vi "controlOutput.vi"(7 "Set":bool, 8 "error in":errorcluster, 9 "enable output in":bool=TRUE, 10 "axis in":u8, 11 "connection ID":refnum<k5>) -> (0 "error out":errorcluster, 1 "enable output out":bool=TRUE, 2 "axis out":u8, 3 "connection ID":refnum<k5>)   [LabVIEW 2019]
panel:
  in  "Set Command":string="com.attocube.amc.control.setControlOutput"
  in  "Get Command":string="com.attocube.amc.control.getControlOutput"
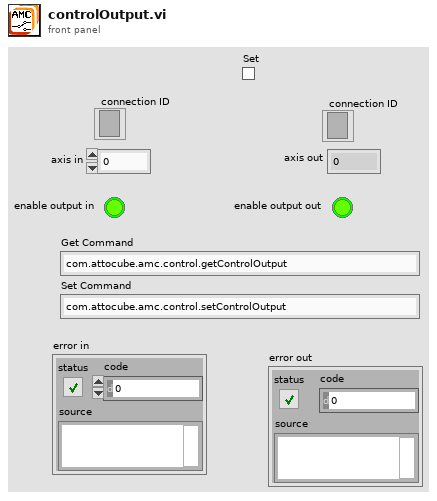
[diagram p1: front panel]
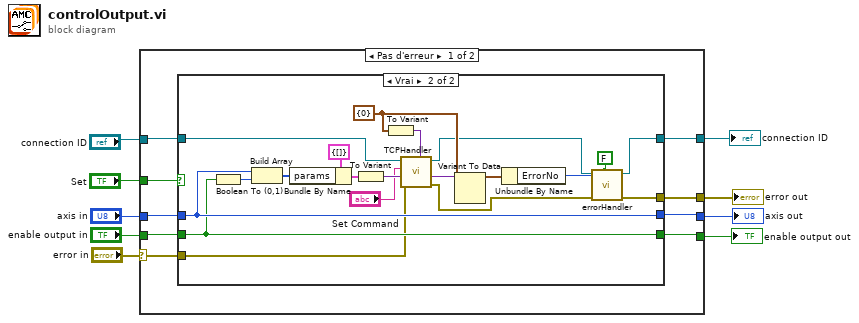
[diagram p0: block diagram]
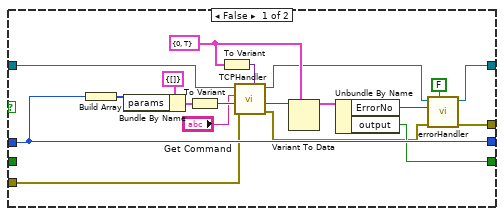
[diagram p2: hidden frame]
diagram:
  n1 = case shown="Pas d'erreur" "error in" {
    selector: "error in" -> [w10 w61]
    tunnel: "axis in" -> [w16 w59]
    tunnel: [w11 w61] -> w1
    tunnel: [w15 w59] -> w8
    tunnel: "Set" -> [w12 _]
    tunnel: [w13 w60] -> w6
    tunnel: "enable output in" -> [w14 w60]
    tunnel: [w18 w58] -> w4
    tunnel: "connection ID" -> [w17 w58]
    frame No Error {
      n2 = case shown="Vrai" w12 {
        tunnel: [w22 w41] -> w18
        tunnel: w17 -> [w27 w51]
        tunnel: w16 -> [w29 w49]
        tunnel: [w29 w49] -> w15
        tunnel: [w26 w48] -> w13
        tunnel: w14 -> [_ w48]
        tunnel: [w28 w45] -> w11
        tunnel: w10 -> [w20 w38]
        frame False {
          w24 = cluster{"ErrorNo":i16, "output":bool} {"ErrorNo"=0, "output"=TRUE} ("input cluster")
          n3 = Build Array(w29) -> (w33:u8[])
          n4 = Bundle By Name(cluster=cluster{"params":i32[]} {"params"=[]} ("input cluster"), "params"=w33) -> (w34:cluster{"params":i32[]})
          n5 = To Variant(anything=w34) -> (Variant=w35:variant)
          n6 = To Variant(anything=w24) -> (Variant=w25:variant)
          n7 = call <userlib>:"TCPHandler.vi"("result Types"=w25, "error in (no error)"=w20, "params"=w35, "method"="Get Command", "connection ID"=w27) -> ("error out"=w19:errorcluster, "result"=w31:variant, "connection ID"=w23:refnum<k5>)  [unwired: 3 in, 1 out]
          n8 = Variant To Data(type=w24, Variant=w31) -> (data=w36:cluster{"ErrorNo":i16, "output":bool})  [unwired: 1 in, 1 out]
          n9 = Unbundle By Name(w36) -> ("ErrorNo"=w37:i16, "output"=w26:bool)
          n10 = call <userlib>:"errorHandler.vi"("show popup"=FALSE, "error in"=w19, "error number"=w37, "connection ID"=w23) -> ("error out"=w28:errorcluster, "connection ID"=w22:refnum<k5>)  [unwired: 6 in]
        }
        frame True {
          w43 = cluster{"ErrorNo":i16} {"ErrorNo"=0} ("input cluster")
          n11 = Boolean To (0,1)(Boolean=w48) -> (0, 1=w55:i16)
          n12 = Build Array(w49, w55) -> (w53:i16[])
          n13 = Bundle By Name(cluster=cluster{"params":i32[]} {"params"=[]} ("input cluster"), "params"=w53) -> (w52:cluster{"params":i32[]})
          n14 = To Variant(anything=w52) -> (Variant=w50:variant)
          n15 = To Variant(anything=w43) -> (Variant=w44:variant)
          n16 = call <userlib>:"TCPHandler.vi"("result Types"=w44, "error in (no error)"=w38, "params"=w50, "method"="Set Command", "connection ID"=w51) -> ("error out"=w40:errorcluster, "result"=w56:variant, "connection ID"=w42:refnum<k5>)  [unwired: 3 in, 1 out]
          n17 = Variant To Data(type=w43, Variant=w56) -> (data=w47:cluster{"ErrorNo":i16})  [unwired: 1 in, 1 out]
          n18 = Unbundle By Name(w47) -> ("ErrorNo"=w46:i16)
          n19 = call <userlib>:"errorHandler.vi"("show popup"=FALSE, "error in"=w40, "error number"=w46, "connection ID"=w42) -> ("error out"=w45:errorcluster, "connection ID"=w41:refnum<k5>)  [unwired: 6 in]
        }
      }
    }
    frame Error {
    }
  }
  "error out" <- w1
  "axis out" <- w8
  "enable output out" <- w6
  "connection ID" <- w4
